vi "Thermal Chamber Controller with DUT.vi"() -> ()   [LabVIEW 2015]
doc: "Implements a Thermal Chamber Controller with a single DUT, using a <b>singleton</b> Delacor QMH Module for the controller, and a single instance of a <b>cloneable</b> Delacor QMH module for the DUT. The chamber is configured to reach a temperature set point. Once the temperature is reached, the Unit Under Test (UUT) performs a Self Test and returns the result. The Unit Under Test code is configured for an 80% pass rate for demonstration purposes.\n\nThis example illustrates that there is no need to have an event structure in the calling code and provides an example of two DQMH modules being used in a traditional \"Configure > Read/Write > Close\" application.\n____\nDelacor QMH Thermal Chamber Examples 4.0.0.21\nCopyright (c) 2018, Delacor"
uses:
  Libraries/Thermal Chamber Controller_DQMH/Heater State--enum.ctl
  Libraries/Thermal Chamber Controller_DQMH/Thermal Chamber Controller_DQMH.lvlib
  Libraries/Device Under Test_Cloneable_DQMH/Device Under Test_Cloneable_DQMH.lvlib
panel:
  out "Self Test Result":bool
  # "Overview: Demonstrates how to implement a Thermal Chamber Controller with a single DUT, using a singleton Delacor QMH Module for the controller, and a single instance of a cloneable Delacor QMH module for the DUT.\nRequirements: Delacor QMH\nInstructions:\n1. Make sure you are already familiar with the concepts described in the Thermal Chamber Controller.vi example in the DQMH Fundamentals project.\n2. Run this VI to launch the singleton Thermal Chamber Controller DQMH module and a single instance of the Device Under Test DQMH module.\n3. Observe the temperature in the Thermal Chamber rise as it approaches the set point.\n4. Once the temperature has been reached, observe that the DUT test simulation starts.\n5. Once the DUT test is complete, the example will stop. See the block diagram of this VI for more information."
  # "(The DUT simulator has a self test pass rate of 80%)."
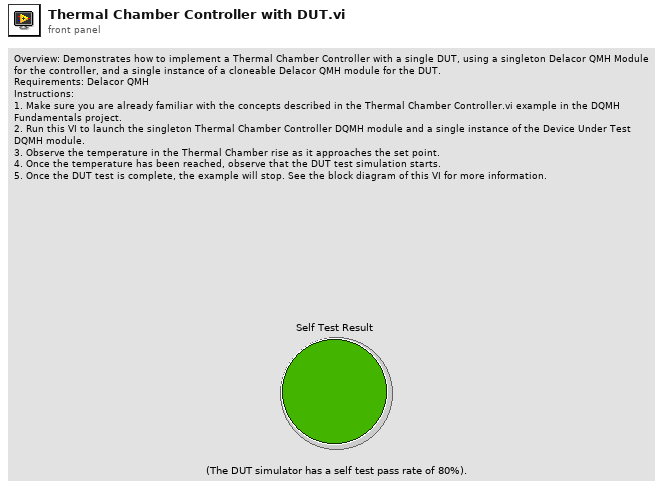
[diagram p1: front panel]
types:
  T1 = typedef "Thermal Chamber Controller_DQMH.lvlib/Heater State--enum.ctl" = enum16{"Heater Enabled", "Heater Disabled"}
  T2 = typedef "Thermal Chamber Controller_DQMH.lvlib/Request and Wait for Status (Reply Payload)--cluster.ctl" = cluster{"Actual Temperature":dbl, "Temperature Set Point":dbl, "Temperature Ramp Rate":dbl, "Heater State":T1, "error":errorcluster}
  T3 = typedef "Device Under Test_Cloneable_DQMH.lvlib/Perform Self Test (Reply Payload)--cluster.ctl" = cluster{"Result":bool, "error":errorcluster}
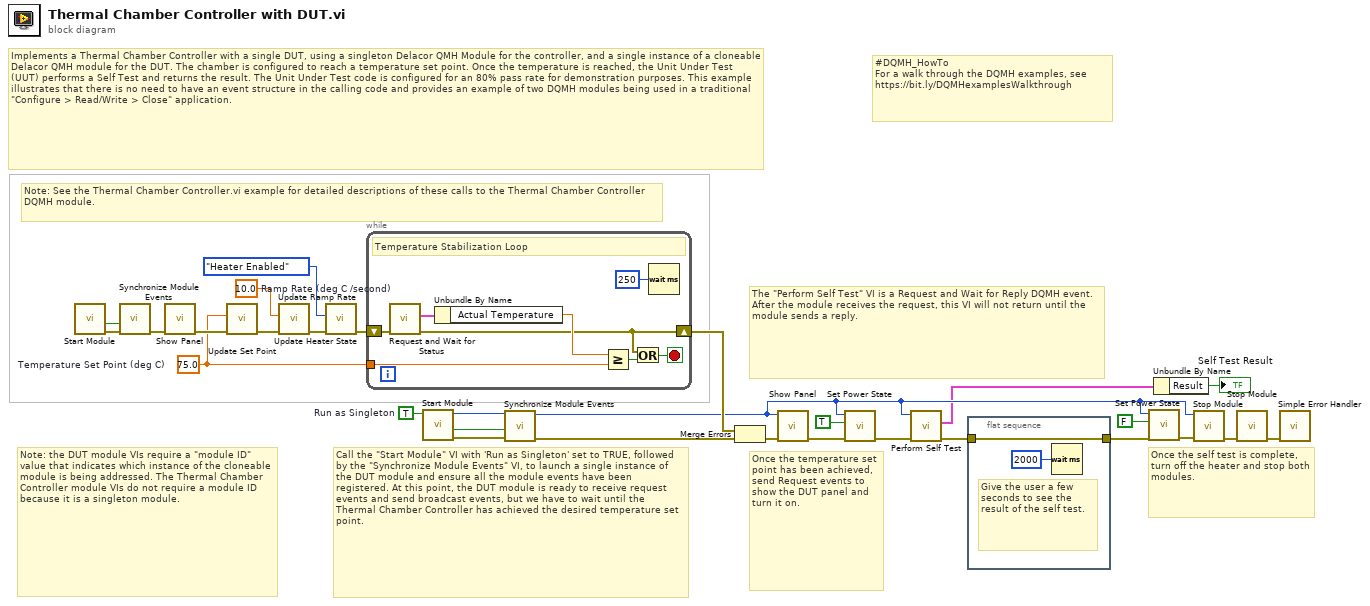
[diagram p0: block diagram]
diagram:
  w1 = TRUE  # Run as Singleton
  w21 = 10.0  # Ramp Rate (deg C /second)
  w20 = 75.0  # Temperature Set Point (deg C)
  # "#DQMH_HowTo \nFor a walk through the DQMH examples, see https://bit.ly/DQMHexamplesWalkthrough"
  # "Note: the DUT module VIs require a \"module ID\" value that indicates which instance of the cloneable module is being addressed. The Thermal Chamber Controller module VIs do not require a module ID because it is a singleton module."
  # "Once the temperature set point has been achieved, send Request events to show the DUT panel and turn it on."
  # "Once the self test is complete, turn off the heater and stop both modules."
  # "Call the \"Start Module\" VI with 'Run as Singleton' set to TRUE, followed by the \"Synchronize Module Events\" VI, to launch a single instance of the DUT module and ensure all the module events have been registered. At this point, the DUT module is ready to receive request events and send broadcast events, but we have to wait until the Thermal Chamber Controller has achieved the desired temperature set point."
  # "Note: See the Thermal Chamber Controller.vi example for detailed descriptions of these calls to the Thermal Chamber Controller DQMH module."
  # "Implements a Thermal Chamber Controller with a single DUT, using a singleton Delacor QMH Module for the controller, and a single instance of a cloneable Delacor QMH module for the DUT. The chamber is configured to reach a temperature set point. Once the temperature is reached, the Unit Under Test (UUT) performs a Self Test and returns the result. The Unit Under Test code is configured for an 80% pass rate for demonstration purposes. This example illustrates that there is no need to have an event structure in the calling code and provides an example of two DQMH modules being used in a traditional \"Configure > Read/Write > Close\" application."
  # "The \"Perform Self Test\" VI is a Request and Wait for Reply DQMH event. After the module receives the request, this VI will not return until the module sends a reply."
  n1 = call "Start Module.vi"() -> ("error out"=w25:errorcluster, "Wait for Event Sync?"=w22:bool)  [unwired: 8 in, 2 out]
  n2 = call "Synchronize Module Events.vi"("error in (no error)"=w25, "Wait for Event Sync?"=w22) -> ("error out"=w24:errorcluster)  [unwired: 9 in]
  n3 = call "Show Panel.vi"("error in (no error)"=w24) -> ("error out"=w23:errorcluster)  [unwired: 10 in]
  n4 = call "Update Set Point.vi"("error in (no error)"=w23, "Temperature Set Point"=w20) -> ("error out"=w27:errorcluster)  [unwired: 9 in]
  n5 = call "Update Ramp Rate.vi"("error in (no error)"=w27, "Temperature Ramp Rate"=w21) -> ("error out"=w26:errorcluster)  [unwired: 9 in]
  n6 = call "Update Heater State.vi"("error in (no error)"=w26, "Heater State"=Heater_State--enum."Heater Enabled") -> ("error out"=w29:errorcluster)  [unwired: 9 in]
  n7 = while {
    shift-right: [w30] -> w19
    shift-left: w29 -> [w34]
    tunnel: w20 -> [w37]
    stop <- w31 stop-if-true
    # "Temperature Stabilization Loop"
    n8 = call "Request and Wait for Status.vi"("error in (no error)"=w34) -> ("error out"=w30:errorcluster, "Reply Payload"=w33:T2)  [unwired: 8 in, 1 out]
    n9 = Unbundle By Name(w33) -> ("Actual Temperature"=w35:dbl)
    n10 = Greater Or Equal?(x=w35, y=w37) -> (x >= y?=w36:bool)
    n11 = Or(x=w30, y=w36) -> (x .or. y?=w31:bool)
    n12 = Wait (ms)(milliseconds to wait=u32 250) -> ()  [unwired: 1 out]
  }
  n13 = call "Start Module.vi"("Run as Singleton? (F)"=w1) -> ("error out"=w17:errorcluster, "Wait for Event Sync?"=w18:bool, "Module ID"=w16:i32)  [unwired: 7 in, 1 out]
  n14 = call "Synchronize Module Events.vi"("error in (no error)"=w17, "Wait for Event Sync?"=w18, "Module ID"=w16) -> ("error out"=w15:errorcluster, "Module ID (dup)"=w11:i32)  [unwired: 7 in]
  n15 = Merge Errors(w19, w15) -> (w7:errorcluster)
  n16 = call "Show Panel.vi"("error in (no error)"=w7, "Module ID"=w11) -> ("error out"=w10:errorcluster)  [unwired: 9 in]
  n17 = call "Set Power State.vi"("error in (no error)"=w10, "Power State"=TRUE, "Module ID"=w11) -> ("error out"=w9:errorcluster)  [unwired: 8 in]
  n18 = call "Perform Self Test.vi"("error in (no error)"=w9, "Module ID"=w11) -> ("error out"=w8:errorcluster, "Reply Payload"=w5:T3)  [unwired: 7 in, 1 out]
  n19 = flat-sequence {
    tunnel: w8 -> [w39]
    tunnel: [w39] -> w14
    frame #0 {
      # "Give the user a few seconds to see the result of the self test."
      n20 = Wait (ms)(milliseconds to wait=u32 2000) -> ()  [unwired: 1 out]
    }
  }
  n21 = call "Set Power State.vi"("error in (no error)"=w14, "Power State"=FALSE, "Module ID"=w11) -> ("error out"=w13:errorcluster)  [unwired: 8 in]
  n22 = Unbundle By Name(w5) -> ("Result"=→"Self Test Result":bool)
  n23 = call "Stop Module.vi"("error in (no error)"=w13, "Module ID"=w11) -> ("error out"=w12:errorcluster)  [unwired: 9 in]
  n24 = call "Stop Module.vi"("error in (no error)"=w12) -> ("error out"=w28:errorcluster)  [unwired: 10 in]
  n25 = call <vilib>:"Simple Error Handler.vi"("error in (no error)"=w28) -> ()  [unwired: 4 in, 5 out]
